vi "txtFile to Excel.vi"   [LabVIEW 2017]
uses:
  <vilib>/addons/_office/excel.llb/Excel Easy Table (str).vi
  <vilib>/Utility/NIReport.llb/NI_report.lvclass
  <vilib>/addons/_office/NI_ReportGenerationToolkit.lvlib
types:
  T1 = enum16{"Standard Report", "HTML", "Word", "Excel"}
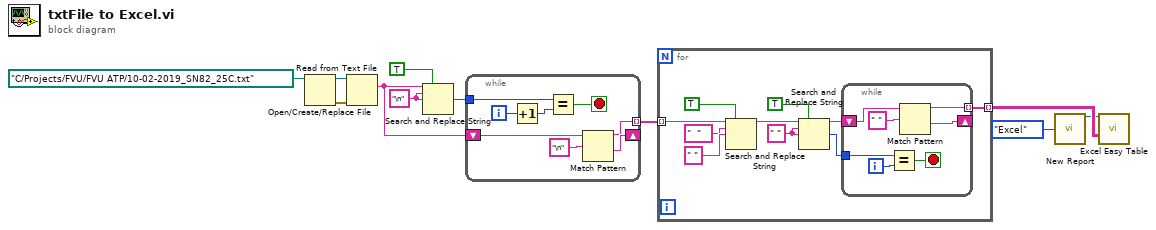
[diagram p0: block diagram]
diagram:
  w7 = "\n" ("regular expression")
  n1 = Open/Create/Replace File(file path (use dialog)=path "C:/Projects/FVU/FVU ATP/10-02-2019_SN82_25C.txt") -> (refnum out=w9:refnum<file>, error out=w11:errorcluster)  [unwired: 5 in, 1 out]
  n2 = Read from Text File(file (use dialog)=w9, error in=w11) -> (text=w8:string)  [unwired: 2 in, 3 out]
  n3 = Search and Replace String(replace all?=TRUE ("replace all? (F)"), input string=w8, search string=w7, replace string=w7) -> (number of replacements=w6:i32)  [unwired: 4 in, 3 out]
  n4 = while {
    shift-right: [w17] -> _
    shift-left: w8 -> [w19]
    tunnel: [w16] -> w4 mode=indexing
    tunnel: w6 -> [w15]
    i -> [w14]
    stop <- w12 stop-if-true
    n5 = Increment(x=w14) -> (x+1=w13:i32)
    n6 = Equal?(x=w15, y=w13) -> (x = y?=w12:bool)
    n7 = Match Pattern(string=w19, regular expression="\n") -> (before substring=w16:string, after substring=w17:string)  [unwired: 1 in, 2 out]
  }
  n8 = for {
    tunnel: w4 -> [w23] mode=indexing
    tunnel: [w26] -> w2 mode=indexing
    w27 = " " ("regular expression")
    n9 = Search and Replace String(replace all?=TRUE ("replace all? (F)"), input string=w23, search string="  " ("regular expression"), replace string=" " ("regular expression")) -> (result string=w22:string)  [unwired: 4 in, 3 out]
    n10 = Search and Replace String(replace all?=TRUE ("replace all? (F)"), input string=w22, search string=w27, replace string=w27) -> (result string=w20:string, number of replacements=w28:i32)  [unwired: 4 in, 2 out]
    n11 = while {
      shift-right: [w34] -> _
      shift-left: w20 -> [w36]
      tunnel: [w33] -> w26 mode=indexing
      tunnel: w28 -> [w32]
      i -> [w30]
      stop <- w31 stop-if-true
      n12 = Equal?(x=w32, y=w30) -> (x = y?=w31:bool)
      n13 = Match Pattern(string=w36, regular expression=" ") -> (before substring=w33:string, after substring=w34:string)  [unwired: 1 in, 2 out]
    }
  }
  n14 = call <vilib>:"New Report.vi"("report type"=T1."Excel") -> ("report out"=w1:refnum<class "NI_report.lvclass">)  [unwired: 13 in, 1 out]
  n15 = call-poly <vilib>:"Excel Easy Table.vi"("report in"=w1, "text data"=w2) -> ()  [unwired: 9 in, 5 out]
